vi "Write SerialConfig.vi"(8 "error in (no error)":errorcluster, 10 "Serial":T1={"Serial Protocol"=enum."RS485", "Protocol Parameters"={"VISA resource name"="", "Baud Rate"=9600, "Data Bits"=8, "Parity"=enum."None", "Flow Control"=0, "Stop Bits"=10, "Timeout (ms)"=10000}, "Serial Message Parameters"={"Byte Count"=200, "Enable Termination Character"=FALSE, "Termination Char"=200}} {"Serial Message Parameters"."Termination Char" format="%x"; "Protocol Parameters"."Stop Bits" items=["1.0"=10, "1.5"=15, "2.0"=20]; "Protocol Parameters"."Flow Control" items=["None", "XON/XOFF", "RTS/CTS", "XON/XOFF & RTS/CTS", "DTR/DSR", "XON/XOFF & DTR/DSR"]; "Protocol Parameters"."Data Bits" min=5 max=8 step=1}, 11 "SerialCommunication in":refnum<class "SerialCommunication.lvclass">) -> (0 "error out":errorcluster, 3 "SerialCommunication out":refnum<class "SerialCommunication.lvclass">)   [LabVIEW 2016, in "SerialCommunication.lvclass"]
uses:
  SerialCommunication.lvclass
  common_serialprotocols/Configuration/SerialConfig.ctl
  common_serialprotocols/Configuration/SerialProtocol.ctl
  common_serialprotocols/Configuration/ProtocolParameters.ctl
  common_serialprotocols/Configuration/SerialMessageParameters.ctl
  SerialCommunication.lvclass/SerialCommunication.ctl
  common_serialprotocols/SerialProtocols.lvlib
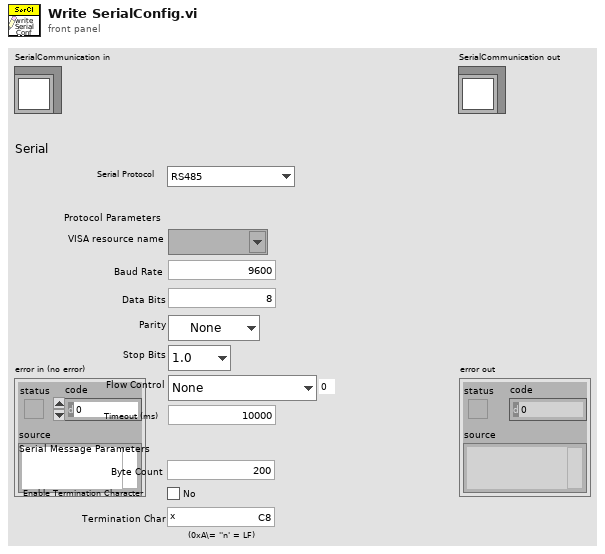
[diagram p1: front panel]
types:
  T1 = typedef "SerialProtocols.lvlib/SerialConfig.ctl" = cluster{"Serial Protocol":T2, "Protocol Parameters":T3, "Serial Message Parameters":T4}
  T2 = typedef "SerialProtocols.lvlib/SerialProtocol.ctl" = enum16{"RS232", "RS485", "SerialSimulator"}
  T3 = typedef "SerialProtocols.lvlib/ProtocolParameters.ctl" = cluster{"VISA resource name":refnum<visa-resource-name>, "Baud Rate":u32, "Data Bits":u16, "Parity":enum16{"None", "Odd", "Even", "Mark", "Space"}, "Flow Control":u16, "Stop Bits":u16, "Timeout (ms)":u32}
  T4 = typedef "SerialProtocols.lvlib/SerialMessageParameters.ctl" = cluster{"Byte Count":u32, "Enable Termination Character":bool, "Termination Char":u8}
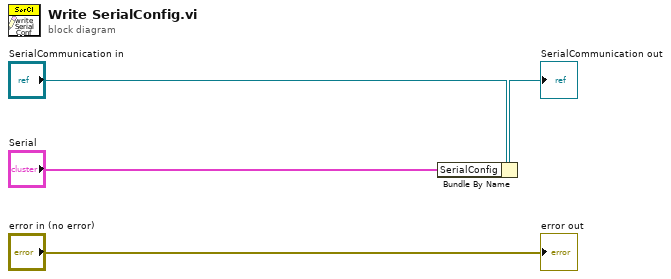
[diagram p0: block diagram]
diagram:
  n1 = Bundle By Name(cluster="SerialCommunication in", "SerialConfig"="Serial") -> (→"SerialCommunication out":refnum<class "SerialCommunication.lvclass">)
  "error out" <- "error in (no error)"
